vi "Orca Flash Filename Proof.vi"(11 "Input Path":path=path "C:/Users/4PiSMS/Desktop/junk/junk_0004_COPY_0") -> (3 "Output path":path)   [LabVIEW 2025]
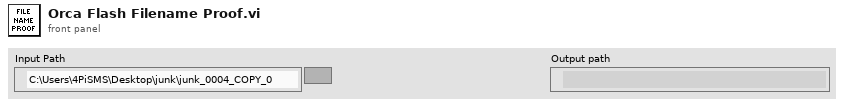
[diagram p1: front panel]
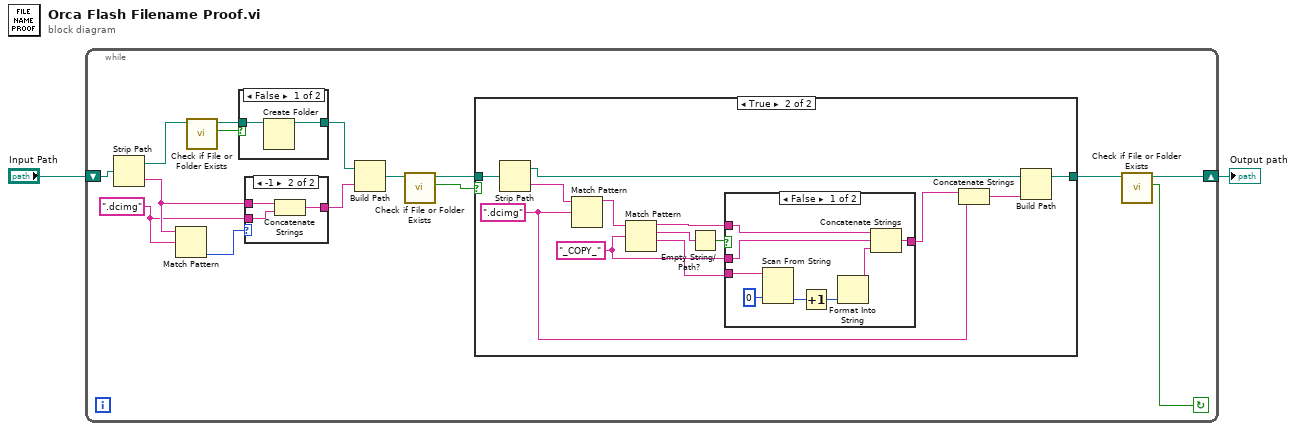
[diagram p0: block diagram]
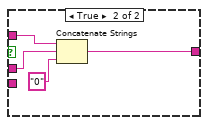
[diagram p4: hidden frame]
diagram:
  n1 = while {
    shift-right: [w7] -> w1
    shift-left: "Input Path" -> [w16]
    stop <- w8 continue-if-true
    w13 = ".dcimg" ("string")
    n2 = Strip Path(path=w16) -> (stripped path=w6:path, name=w14:string)
    n3 = Match Pattern(string=w14, regular expression=w13) -> (offset past match=w12:i32)  [unwired: 1 in, 3 out]
    n4 = call <vilib>:"Check if File or Folder Exists.vi"("path"=w6) -> ("file or folder exists?"=w5:bool, "dup path"=w4:path)  [unwired: 8 in, 1 out]
    n5 = case shown="False" w5 {
      tunnel: [w18 w20] -> w3
      tunnel: w4 -> [w19 w20]
      frame False {
        n6 = Create Folder(path (use dialog)=w19) -> (created path=w18:path)  [unwired: 2 in, 2 out]
      }
      frame True {
      }
    }
    n7 = case shown="-1" w12 {
      tunnel: [w47 w50] -> w15
      tunnel: w14 -> [w47 w49]
      tunnel: w13 -> [_ w48]
      frame 0, Default {
      }
      frame -1 {
        n8 = Concatenate Strings(w49, w48) -> (w50:string)
      }
    }
    n9 = Build Path(base path=w3, name or relative path=w15) -> (appended path=w17:path)
    n10 = call <vilib>:"Check if File or Folder Exists.vi"("path"=w17) -> ("file or folder exists?"=w11:bool, "dup path"=w10:path)  [unwired: 8 in, 1 out]
    n11 = case shown="True" w11 {
      tunnel: [w21 w26] -> w9
      tunnel: w10 -> [w21 w34]
      frame False {
      }
      frame True {
        w27 = "_COPY_"
        w22 = ".dcimg"
        n12 = Strip Path(path=w34) -> (stripped path=w32:path, name=w33:string)
        n13 = Match Pattern(string=w33, regular expression=w22) -> (before substring=w31:string)  [unwired: 1 in, 3 out]
        n14 = Match Pattern(string=w31, regular expression=w27) -> (before substring=w28:string, match substring=w30:string, after substring=w24:string)  [unwired: 1 in, 1 out]
        n15 = Empty String/Path?(string/path=w30) -> (empty?=w29:bool)
        n16 = case shown="False" w29 {
          tunnel: w28 -> [w40 w46]
          tunnel: w27 -> [w39 w45]
          tunnel: [w37 w43] -> w25
          tunnel: w24 -> [w42 _]
          frame False {
            n17 = Scan From String(input string=w42, default 1=0) -> (output 1=w41:i32)  [unwired: 3 in, 3 out]
            n18 = Increment(x=w41) -> (x+1=w35:i32)
            n19 = Format Into String(w35) -> (resulting string=w38:string)  [unwired: 3 in, 1 out]
            n20 = Concatenate Strings(w40, w39, w38) -> (w37:string)
          }
          frame True {
            n21 = Concatenate Strings(w46, w45, "0" ("string")) -> (w43:string)
          }
        }
        n22 = Concatenate Strings(w25, w22) -> (w23:string)
        n23 = Build Path(base path=w32, name or relative path=w23) -> (appended path=w26:path)
      }
    }
    n24 = call <vilib>:"Check if File or Folder Exists.vi"("path"=w9) -> ("file or folder exists?"=w8:bool, "dup path"=w7:path)  [unwired: 8 in, 1 out]
  }
  "Output path" <- w1
